vi "sub_strain-nulling-old.vi"(8 "error in":errorcluster caption="에러 입력") -> (0 "error out":errorcluster caption="에러 출력", 3 "offset":T1)   [LabVIEW 2013]
uses:
  <vilib>/DAQmx/read.llb/DAQmx Read (Analog 1D Wfm NChan NSamp).vi
  <vilib>/measure/madcrms.llb/Basic Averaged DC-RMS for 1 Chan.vi
  <vilib>/DAQmx/miscellaneous.llb/DAQmx Fill In Error Info.vi
  <vilib>/measure/NI_MAPro.lvlib
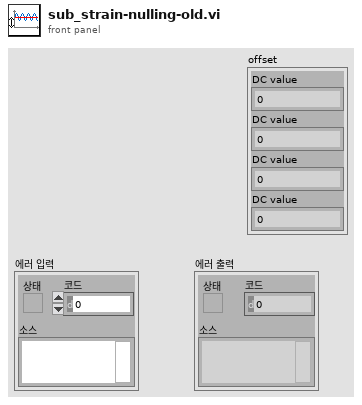
[diagram p1: front panel]
types:
  T1 = cluster{"DC value":dbl, "DC value":dbl, "DC value":dbl, "DC value":dbl}
  T2 = typedef "config_ctl.ctl" = cluster{"Trigger minlevel":dbl, "Lower Cut-Off":dbl, "Force high_level":dbl, "state settings":cluster{"method":enum32{"histogram", "peak", "auto select"}, "histogram size":i32, "histogram method":enum16{"mode"}, "reserved":dbl}}
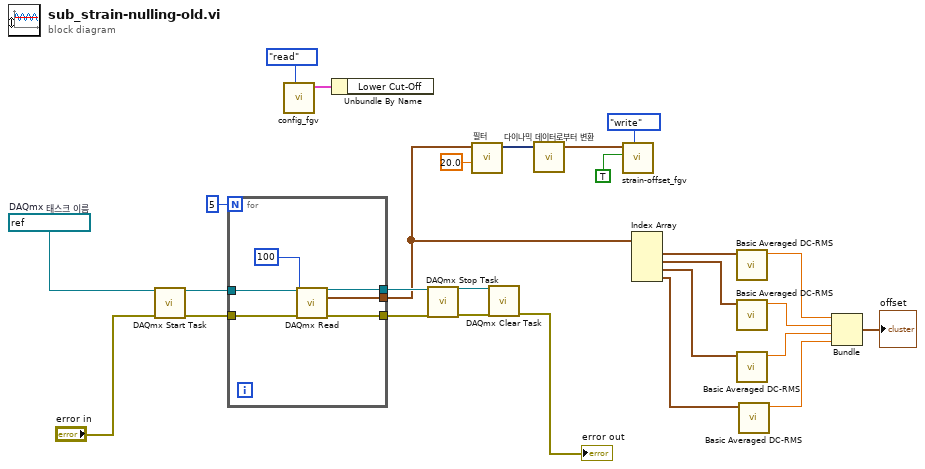
[diagram p0: block diagram]
diagram:
  w27 = refnum<k21> "9237_0327"  # DAQmx 태스크 이름
  n1 = call <vilib>:"DAQmx Start Task.vi"("task/channels in"=w27, "error in"="error in") -> ("task out"=w25:refnum<k21>, "error out"=w26:errorcluster)  [unwired: 12 in]
  n2 = for {
    N: 5 -> [_]
    tunnel: w26 -> [w32]
    tunnel: w25 -> [w31]
    tunnel: [w30] -> w22
    tunnel: [w29] -> w21
    tunnel: [w28] -> w6
    n3 = call-poly <vilib>:"DAQmx Read.vi"("task/channels in"=w31, "number of samples per channel"=100, "error in"=w32) -> ("task out"=w29:refnum<k21>, "data"=w28:waveform(dbl)[], "error out"=w30:errorcluster)  [unwired: 10 in]
  }
  n4 = call "config_fgv.vi"("cmd"=enum16{"write", "read", "ini"}."read") -> ("Config out"=w5:T2)  [unwired: 9 in, 1 out]
  n5 = Unbundle By Name(w5) -> ()  [unwired: 1 out]
  n6 = call <vilib>:"DAQmx Stop Task.vi"("task/channels in"=w21, "error in"=w22) -> ("task out"=w23:refnum<k21>, "error out"=w24:errorcluster)  [unwired: 12 in]
  n7 = call "필터"("Lower Cut-Off"=20.0, "Signal"=w6) -> ("Filtered Signal"=w3:dynamicdata)  [unwired: 8 in, 1 out]
  n8 = call <vilib>:"DAQmx Clear Task.vi"("task in"=w23, "error in"=w24) -> ("error out"=→"error out":errorcluster)  [unwired: 13 in]
  n9 = call "다이나믹 데이터로부터 변환"("Dynamic Data Type"=w3) -> ("Array of Waveform"=w2:waveform(dbl)[])  [unwired: 3 in]
  n10 = call "strain-offset_fgv.vi"("cmd"=enum16{"write", "read"}."write" ("열거형"), "input?"=TRUE, "data"=w2) -> ()  [unwired: 8 in, 1 out]
  n11 = Index Array(array=w6) -> (element #1=w16:waveform(dbl), element #2=w15:waveform(dbl), element #3=w14:waveform(dbl), element #4=w13:waveform(dbl))  [unwired: 4 in]
  n12 = call-poly <vilib>:"Basic Averaged DC-RMS.vi"("signal in"=w16) -> ("DC value"=w12:dbl)  [unwired: 7 in, 3 out]
  n13 = call-poly <vilib>:"Basic Averaged DC-RMS.vi"("signal in"=w15) -> ("DC value"=w11:dbl)  [unwired: 7 in, 3 out]
  n14 = call-poly <vilib>:"Basic Averaged DC-RMS.vi"("signal in"=w14) -> ("DC value"=w10:dbl)  [unwired: 7 in, 3 out]
  n15 = call-poly <vilib>:"Basic Averaged DC-RMS.vi"("signal in"=w13) -> ("DC value"=w9:dbl)  [unwired: 7 in, 3 out]
  n16 = Bundle("DC value"=w12, "DC value"=w11, "DC value"=w10, "DC value"=w9) -> (→"offset":T1)  [unwired: 1 in]
